vi "eventSettingsApplied.vi"(8 "error in (no error)":errorcluster, 11 "Publisher in":refnum<class "Publisher.lvclass">) -> (0 "error out":errorcluster, 3 "Publisher out":refnum<class "Publisher.lvclass">)   [LabVIEW 2016, in "Publisher.lvclass"]
uses:
  Publisher.lvclass
  Publisher.lvclass/Publisher.ctl
  Communicator/M1M3SAL/M1M3SAL.lvclass/M1M3SAL.ctl
  Communicator/M1M3SAL/writeHeader.vi
  Communicator/M1M3SAL/writeDBL.vi
  Communicator/M1M3SAL/writeString.vi
  Communicator/M1M3SAL/writeI32.vi
  Communicator/M1M3SAL/writeU8.vi
  Communicator/M1M3SAL/writeU8Array.vi
  Communicator/M1M3SAL/M1M3SAL.lvclass
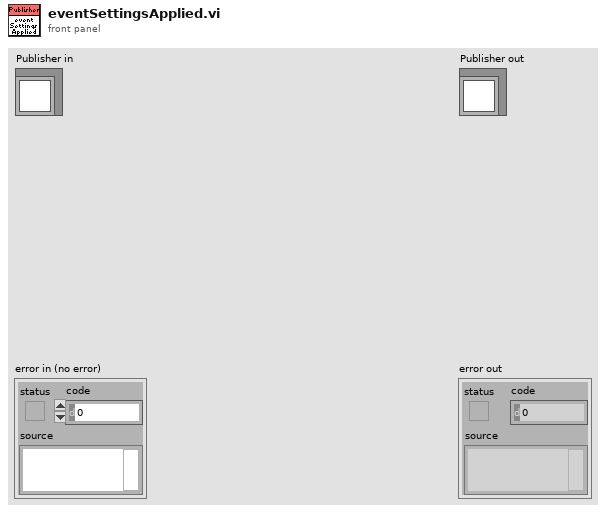
[diagram p1: front panel]
types:
  T1 = typedef "M1M3SupportTopics.lvlib/EventSettingsApplied.ctl" = cluster{"Timestamp":T2, "Settings":string}
  T2 = typedef "M1M3SupportTopics.lvlib/Timestamp.ctl" = dbl
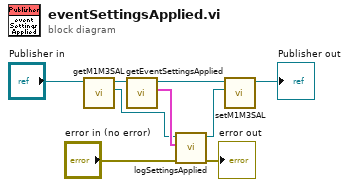
[diagram p0: block diagram]
diagram:
  n1 = call "getM1M3SAL.vi"("Publisher in"="Publisher in") -> ("M1M3SAL"=w4:refnum<class "M1M3SAL.lvclass">, "Publisher out"=w7:refnum<class "Publisher.lvclass">)  [unwired: 9 in]
  n2 = call "getEventSettingsApplied.vi"("Publisher in"=w7) -> ("EventSettingsApplied"=w5:T1, "Publisher out"=w6:refnum<class "Publisher.lvclass">)  [unwired: 9 in]
  n3 = call "logSettingsApplied.vi"("error in (no error)"="error in (no error)", "EventSettingsApplied"=w5, "M1M3SAL in"=w4) -> ("error out"=→"error out":errorcluster, "M1M3SAL out"=w3:refnum<class "M1M3SAL.lvclass">)  [unwired: 7 in]
  n4 = call "setM1M3SAL.vi"("M1M3SAL"=w3, "Publisher in"=w6) -> ("Publisher out"=→"Publisher out":refnum<class "Publisher.lvclass">)  [unwired: 9 in]
